vi "AMWave.vi"() -> ()   [LabVIEW 2015]
uses:
  <vilib>/imath/engines/lvmath2/RunTimeEngine/NodeEndStatement/NIMS_NodeEndStatement_Output.vi
  <instcachedir>/0/NIMS_NodeEndStatement_Output_53EC0D466D134D7ABD903AC30B43404B.lvgen/NIMS_NodeEndStatement_Output_53EC0D466D134D7ABD903AC30B43404B_001.vi
  <vilib>/imath/engines/lvmath2/RunTimeEngine/ErrorHandling/NIMS_Finalize Error.vi
panel:
  out "Time":dbl[](array[numeric])
  out "Displacement":dbl[](array[numeric])
  out "XY Graph":cluster{dbl[], dbl[]}(graph)
  in  "Amplitude":dbl
  in  "Modulation Frequency":dbl
  in  "Sampling Frequency":dbl
  in  "Number of Samples":dbl
  in  "Signal Frequency":dbl
  # "Digitizing Parameters"
  # "AM Wave"
  # "AM Wave Parameters"
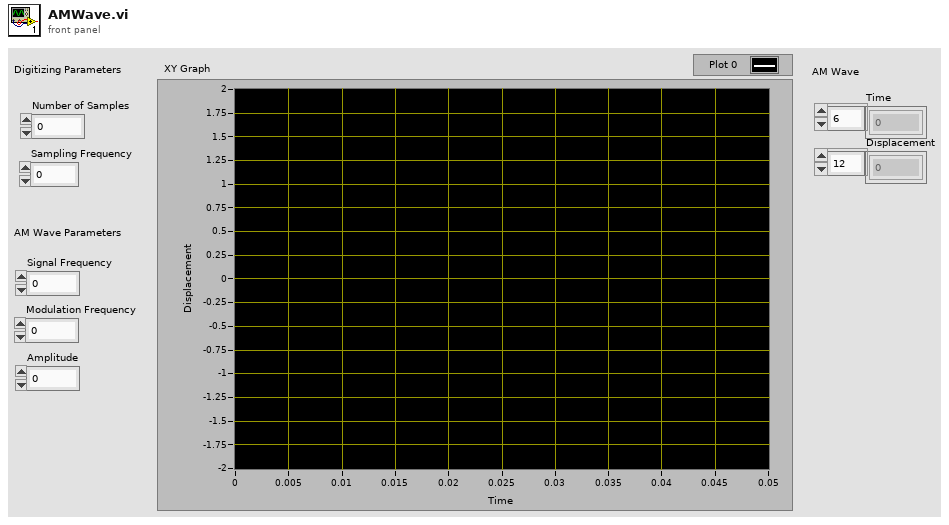
[diagram p1: front panel]
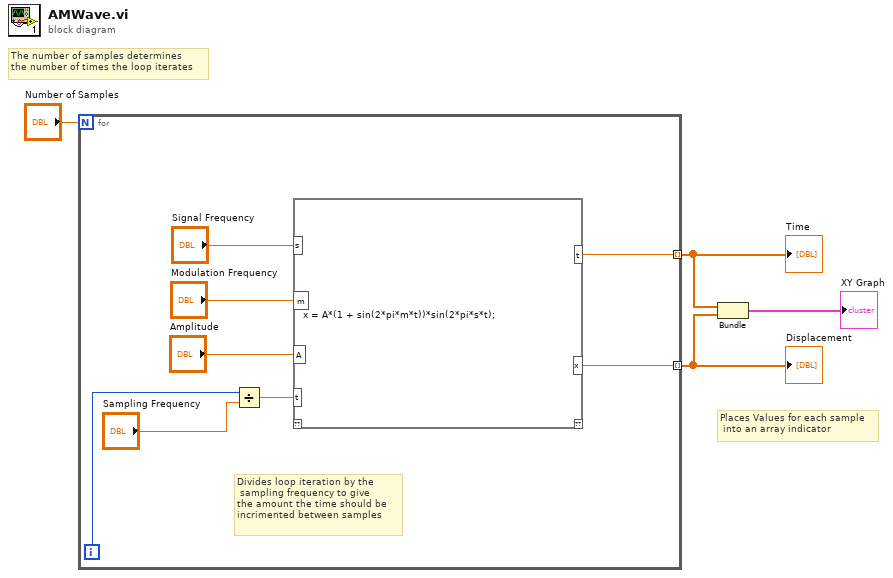
[diagram p0: block diagram]
diagram:
  # "Places Values for each sample\n into an array indicator"
  # "The number of samples determines \nthe number of times the loop iterates"
  n1 = for {
    N: "Number of Samples" -> [_]
    tunnel: [w11] -> w1 mode=indexing
    tunnel: [w10] -> w2 mode=indexing
    i -> [w5]
    # "Equation for AM Wave\nCalculates displacement of\n wave for each point in time"
    # "Divides loop iteration by the\n sampling frequency to give\nthe amount the time should be\nincrimented between samples"
    n2 = Divide(x=w5, y="Sampling Frequency") -> (x/y=w12:dbl)
    n3 = mathscript code="x = A*(1 + sin(2*pi*m*t))*sin(2*pi*s*t);"("s"="Signal Frequency", "t"=w12, "m"="Modulation Frequency", "A"="Amplitude") -> ("x"=w10:dbl, "t"=w11:dbl)  [unwired: 1 in, 1 out]
  }
  "Displacement" <- w2
  "Time" <- w1
  n4 = Bundle(w1, w2) -> (→"XY Graph":cluster{dbl[], dbl[]})  [unwired: 1 in]
